vi "Process DIR.vi"(8 "error in (no error)":errorcluster, 9 "Data > 0":bool, 10 "Data In":string, 11 "Data Cluster in":T1={"Data Display"="", "FP Control Refs"={"Connect to Station Ref"=refnum, "Download Ref"=refnum, "Exit Button Ref"=refnum, "Date Refnum"=refnum, "Path Refnum"=refnum, "COM Port"="", "IP or Phone Ref"=refnum, "TCPIP ID"=refnum, "Reboot Refnum"=refnum}, "FP Indicator Refs"={"Connected Refnum"=refnum, "Data Display Ref"=refnum, "Station ID Ref"=refnum}, "User Events"={"Stop"=refnum, "Update Display"=refnum}, "Message Queues"={"UI"=refnum, "ACQUISITION"=refnum, "PROCESSING"=refnum, "LOGGING"=refnum}, "IS IP?"=FALSE, "DCP Version"=enum."XPert2"}) -> (0 "error out":errorcluster, 3 "Data Cluster out":T1={"Data Display"="", "FP Control Refs"={"Connect to Station Ref"=refnum, "Download Ref"=refnum, "Exit Button Ref"=refnum, "Date Refnum"=refnum, "Path Refnum"=refnum, "COM Port"="", "IP or Phone Ref"=refnum, "TCPIP ID"=refnum, "Reboot Refnum"=refnum}, "FP Indicator Refs"={"Connected Refnum"=refnum, "Data Display Ref"=refnum, "Station ID Ref"=refnum}, "User Events"={"Stop"=refnum, "Update Display"=refnum}, "Message Queues"={"UI"=refnum, "ACQUISITION"=refnum, "PROCESSING"=refnum, "LOGGING"=refnum}, "IS IP?"=FALSE, "DCP Version"=enum."XPert2"})   [LabVIEW 2016]
uses:
  Message Queue/GLDL Message Queue.lvlib
  Great Lakes Downloads/support/Message Queue/Message Queue.lvlib
  Great Lakes Downloads/support/Message Queue/Enqueue Message (Single).vi
  <vilib>/regexp/Match Regular Expression.xnode
  Message Queue/Enqueue Message (Single).vi
  Message Queue/Message Cluster.ctl
  Message Queue/All Message Queues.ctl
  controls/Connected Indicator.ctl
  controls/Output Indicator.ctl
  controls/Disconnect Control.ctl
  controls/Download Control.ctl
  controls/Exit Control.ctl
  controls/Date Control.ctl
  controls/Save Path Control.ctl
  controls/IP Phone Number Control.ctl
  controls/GLDL UI Data.ctl
  controls/Station ID Indicator.ctl
  controls/Reboot Control.ctl
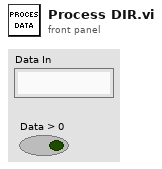
[diagram p1: front panel]
types:
  T1 = typedef "GLDL UI Data.ctl" = cluster{"Data Display":string, "FP Control Refs":cluster{"Connect to Station Ref":refnum<vi>, "Download Ref":refnum<vi>, "Exit Button Ref":refnum<vi>, "Date Refnum":refnum<vi>, "Path Refnum":refnum<vi>, "COM Port":refnum<visa-resource-name>, "IP or Phone Ref":refnum<vi>, "TCPIP ID":refnum<k5>, "Reboot Refnum":refnum<vi>}, "FP Indicator Refs":cluster{"Connected Refnum":refnum<vi>, "Data Display Ref":refnum<vi>, "Station ID Ref":refnum<vi>}, "User Events":cluster{"Stop":refnum<user-event>, "Update Display":refnum<user-event>}, "Message Queues":T2, "IS IP?":bool, "DCP Version":enum16{"XPert", "XPert2"}}
  T2 = typedef "GLDL Message Queue.lvlib/All Message Queues.ctl" = cluster{"UI":refnum<queue>, "ACQUISITION":refnum<queue>, "PROCESSING":refnum<queue>, "LOGGING":refnum<queue>}
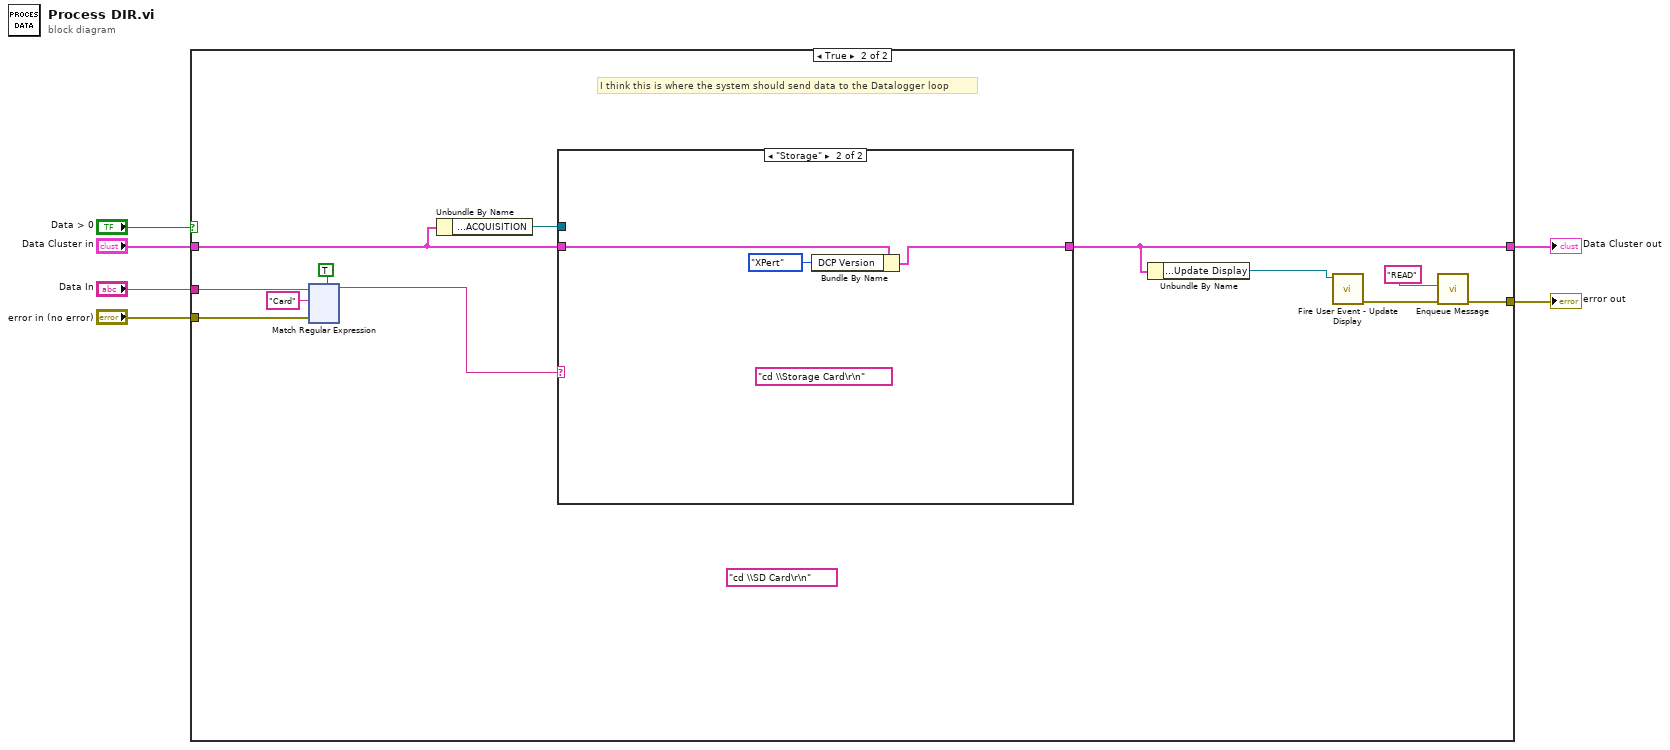
[diagram p0: block diagram]
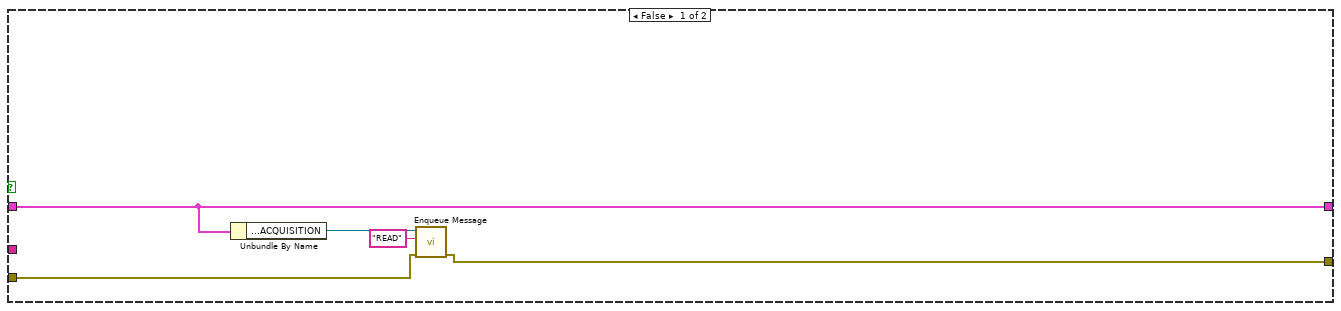
[diagram p2: hidden frame]
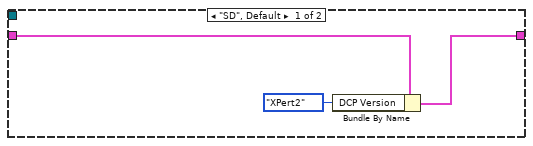
[diagram p3: hidden frame]
diagram:
  n1 = case shown="True" "Data > 0" {
    tunnel: "error in (no error)" -> [w8 w18]
    tunnel: [w7 w22] -> w4
    tunnel: "Data In" -> [_ w20]
    tunnel: "Data Cluster in" -> [w11 w15]
    tunnel: [w11 w13] -> w6
    frame False {
      n2 = Unbundle By Name(w11) -> ("Message Queues.ACQUISITION"=w10:refnum<queue>)
      n3 = call-poly "Enqueue Message.vi"("error in (no error)"=w8, "Message"="READ", "Message Queue"=w10) -> ("error out"=w7:errorcluster)  [unwired: 7 in, 1 out]
    }
    frame True {
      (unwired) "cd \\SD Card\r\n" ("data in")
      # "I think this is where the system should send data to the Datalogger loop"
      n4 = xnode "Match Regular Expression"("input string"=w20, "regular expression"="Card", "error in"=w18, "multiline? (F)"=TRUE) -> ("before match"=w16:string)  [unwired: 2 in, 4 out]
      n5 = Unbundle By Name(w15) -> ("Message Queues.ACQUISITION"=w14:refnum<queue>)
      n6 = case shown="\"Storage\"" w16 {
        tunnel: w15 -> [w25 w27]
        tunnel: [w24 w28] -> w13
        tunnel: w14 -> [_ _]
        frame "SD", Default {
          n7 = Bundle By Name(cluster=w25, "DCP Version"=enum16{"XPert", "XPert2"}."XPert2") -> (w24:T1)
        }
        frame "Storage" {
          (unwired) "cd \\Storage Card\r\n" ("data in")
          n8 = Bundle By Name(cluster=w27, "DCP Version"=enum16{"XPert", "XPert2"}."XPert") -> (w28:T1)
        }
      }
      n9 = Unbundle By Name(w13) -> ("User Events.Update Display"=w12:refnum<user-event>)
      n10 = call "Fire User Event - Update Display.vi"("Update Display"=w12) -> ("error out"=w21:errorcluster)  [unwired: 10 in]
      n11 = call-poly "Enqueue Message.vi"("error in (no error)"=w21, "Message"="READ" ("Initial Message")) -> ("error out"=w22:errorcluster)  [unwired: 8 in, 1 out]
    }
  }
  "Data Cluster out" <- w6
  "error out" <- w4
